vi "returncode.vi"(3 "Return code":i32) -> (0 "Description":string, 1 "retcode":i32)   [LabVIEW 2016]
doc: "Return the description associated with a return code."
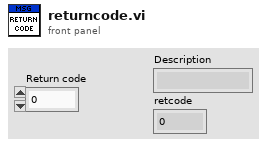
[diagram p1: front panel]
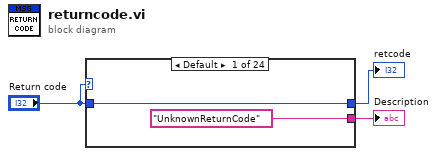
[diagram p0: block diagram]
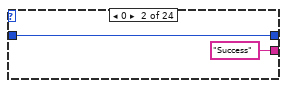
[diagram p2: hidden frame]
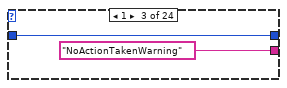
[diagram p3: hidden frame]
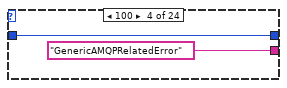
[diagram p4: hidden frame]
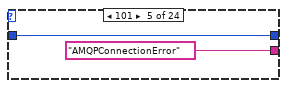
[diagram p5: hidden frame]
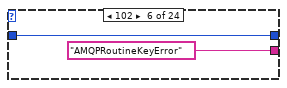
[diagram p6: hidden frame]
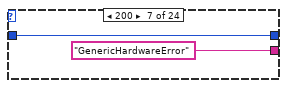
[diagram p7: hidden frame]
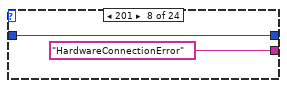
[diagram p8: hidden frame]
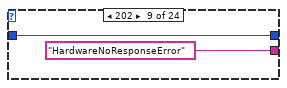
[diagram p9: hidden frame]
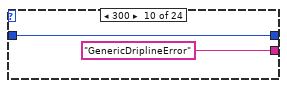
[diagram p10: hidden frame]
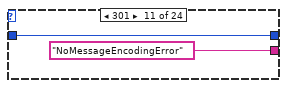
[diagram p11: hidden frame]
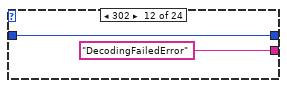
[diagram p12: hidden frame]
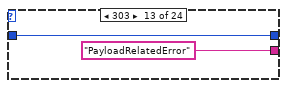
[diagram p13: hidden frame]
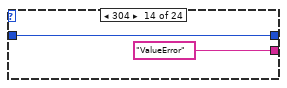
[diagram p14: hidden frame]
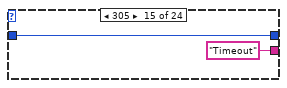
[diagram p15: hidden frame]
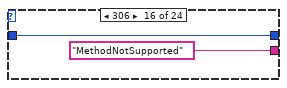
[diagram p16: hidden frame]
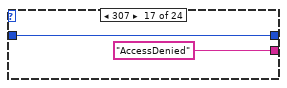
[diagram p17: hidden frame]
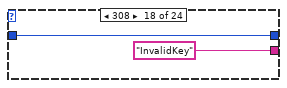
[diagram p18: hidden frame]
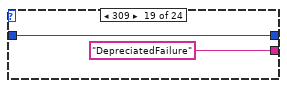
[diagram p19: hidden frame]
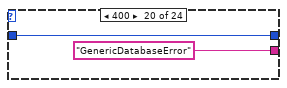
[diagram p20: hidden frame]
diagram:
  n1 = case shown="Default" "Return code" {
    tunnel: ["UnknownReturnCode" "Success" "NoActionTakenWarning" "GenericAMQPRelatedError" "AMQPConnectionError" "AMQPRoutineKeyError" "GenericHardwareError" "HardwareConnectionError" "HardwareNoResponseError" "GenericDriplineError" "NoMessageEncodingError" "DecodingFailedError" "PayloadRelatedError" "ValueError" "Timeout" "MethodNotSupported" "AccessDenied" "InvalidKey" "DepreciatedFailure" "GenericDatabaseError" "GenericDAQError" "DAQNotEnabled" "DAQNotRunning" "UnhandledCoreLanguage"] -> w2
    tunnel: "Return code" -> [w5 w6 w8 w10 w12 w14 w16 w18 w20 w22 w24 w26 w28 w30 w32 w34 w36 w38 w40 w42 w44 w46 w48 w50]
    tunnel: [w5 w6 w8 w10 w12 w14 w16 w18 w20 w22 w24 w26 w28 w30 w32 w34 w36 w38 w40 w42 w44 w46 w48 w50] -> w1
    frame Default {
    }
    frame 0 {
    }
    frame 1 {
    }
    frame 100 {
    }
    frame 101 {
    }
    frame 102 {
    }
    frame 200 {
    }
    frame 201 {
    }
    frame 202 {
    }
    frame 300 {
    }
    frame 301 {
    }
    frame 302 {
    }
    frame 303 {
    }
    frame 304 {
    }
    frame 305 {
    }
    frame 306 {
    }
    frame 307 {
    }
    frame 308 {
    }
    frame 309 {
    }
    frame 400 {
    }
    frame 500 {
    }
    frame 501 {
    }
    frame 502 {
    }
    frame 999 {
    }
  }
  "Description" <- w2
  "retcode" <- w1
